vi "Permit Sleeping.vi"(8 "error in (no error)":errorcluster) -> (0 "error out":errorcluster)   [LabVIEW 2024, in "VIPM Power Requests.lvlib"]
doc: "Permits computer to go to sleep and screen saver to turn on. Actual behavior depends on computer configuration."
uses:
  VIPM Power Requests.lvlib
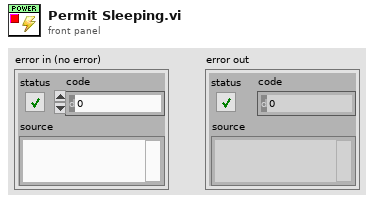
[diagram p1: front panel]
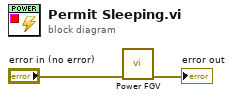
[diagram p0: block diagram]
diagram:
  n1 = call "Power FGV.vi"("error in (no error)"="error in (no error)") -> ("error out"=→"error out":errorcluster)  [unwired: 10 in]
